vi "ReadLidarTesting.vi"() -> ()   [LabVIEW 2014]
uses:
  <instrlib>/Hokuyo URG Series/Public/Initialize-Standard.vi
  <instrlib>/Hokuyo URG Series/Hokuyo URG Series.lvlib
  <vilib>/robotics/Obstacle Avoidance/Advanced Vector Field Histogram/NI_Robotics_Vector Field Histogram.lvlib
panel:
  out "32bit integer":i32
  out "x+y":dbl
  out "x*y":dbl
  in  "maximum heading change (rad)":dbl=1.5707963267948966
  out "Meter":dbl(knob) scale=3.14..-3.14
  out "Waveform Graph":dbl[](graph)
  out "chosen heading (rad)":dbl
  in  "obstacle clearance distance":dbl
  in  "heading":T1
  in  "thresholds":T2
  out "XY Graph":cluster{"X":dbl[], "Y":dbl[]}(graph)
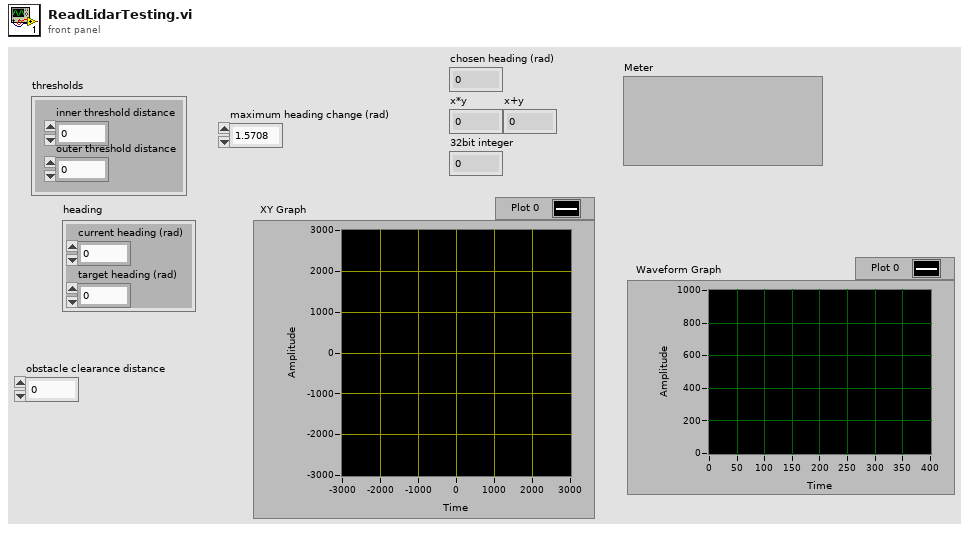
[diagram p1: front panel]
types:
  T1 = cluster{"current heading (rad)":dbl, "target heading (rad)":dbl}
  T2 = cluster{"inner threshold distance":dbl, "outer threshold distance":dbl}
  T3 = cluster{"Magnitude":u16[], "Direction":fxp<+/-,16,8>[]}
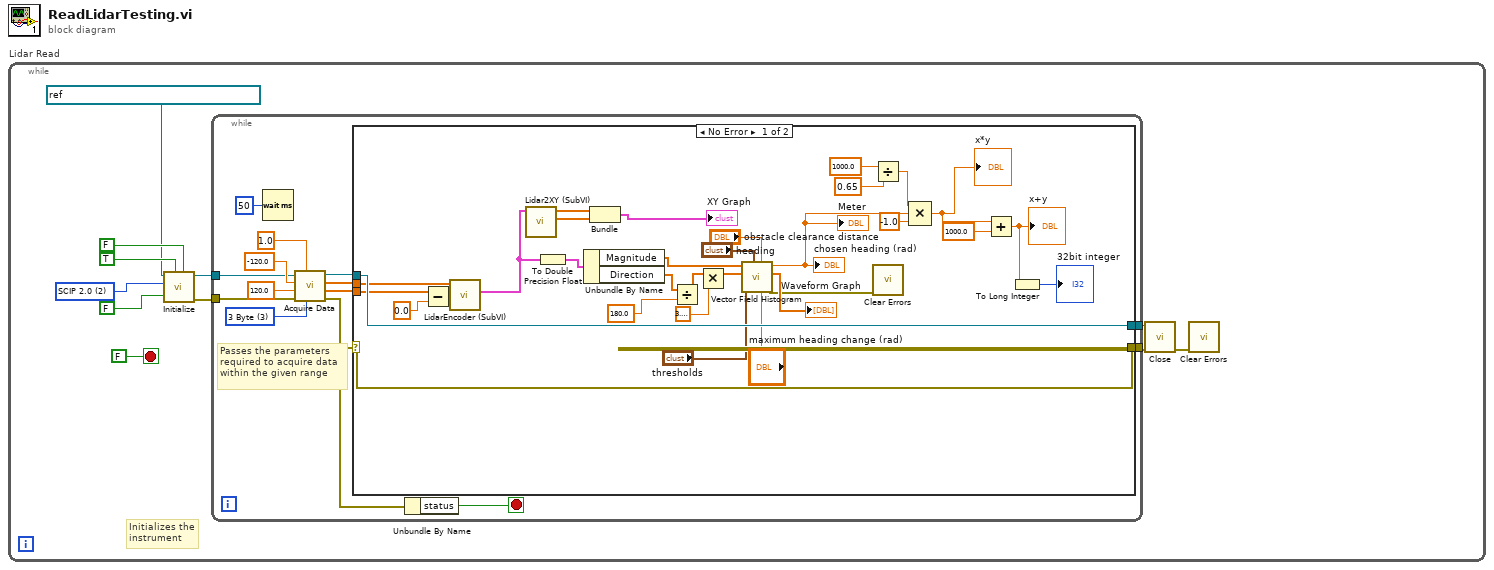
[diagram p0: block diagram]
diagram:
  n1 = while "Lidar Read" {
    stop <- FALSE stop-if-true
    w7 = u32 2 items=["Convert to Latest", "SCIP 1.1", "SCIP 2.0"] ("Protocol")
    # "Initializes the instrument"
    n2 = call-poly <instrlib>:"Initialize.vi"("Reset? (F: No)"=FALSE ("Reset Instrument (Disabled)"), "Checksum (Disabled)"=FALSE ("Checksum"), "ID Query? (Enabled)"=TRUE ("ID Query?"), "Protocol (2: SCIP 2.0)"=w7, "VISA resource name"=refnum<visa-resource-name> "TCPIP::192.168.0.10::10940::SOCKET") -> ("error out"=w4:errorcluster, "VISA resource name out"=w5:refnum<visa-resource-name>)  [unwired: 5 in]
    n3 = while {
      tunnel: w5 -> [w16]
      tunnel: [w25] -> w11
      tunnel: [w24] -> w6
      tunnel: w4 -> [w15]
      stop <- w12 stop-if-true
      w14 = u16 3 items=["2 Byte"=2, "3 Byte"=3] ("Encoding Width")
      # "Passes the parameters\nrequired to acquire data\nwithin the given range"
      n4 = Wait (ms)(milliseconds to wait=u32 50) -> ()  [unwired: 1 out]
      n5 = call <instrlib>:"Acquire Data.vi"("Data Encoding Width (3 Byte)"=w14, "Cluster Count (1)"=1.0 ("Cluster Count"), "error in (no error)"=w15, "End Point (120°)"=120.0 ("End Point"), "Start Point (-120°)"=-120.0 ("Start Point"), "VISA resource name"=w16) -> ("error out"=w20:errorcluster, "Direction"=w21:dbl[], "Magnitude"=w22:dbl[], "VISA resource name out"=w23:refnum<visa-resource-name>)  [unwired: 2 in]
      n6 = case shown="No Error" w20 {
        selector: w20 -> [w56 w59]
        tunnel: [w56 w59] -> w25
        tunnel: w23 -> [w57 w58]
        tunnel: [w57 w58] -> w24
        tunnel: w22 -> [w55 _]
        tunnel: w21 -> [w54 _]
        frame No Error {
          n7 = Subtract(x=w54, y=0.0) -> (x-y=w53:dbl[])
          n8 = call "LidarEncoder (SubVI).vi"("Direction"=w53, "Magnitude"=w55) -> ("Encoded"=w48:T3)  [unwired: 9 in]
          n9 = call "Lidar2XY (SubVI).vi"("Lidar"=w48) -> ("Y"=w50:dbl[], "X"=w51:dbl[])  [unwired: 9 in]
          n10 = To Double Precision Float(number=w48) -> (double precision float=w47:cluster{"Magnitude":dbl[], "Direction":dbl[]})
          n11 = Unbundle By Name(w47) -> ("Magnitude"=w46:dbl[], "Direction"=w44:dbl[])
          n12 = Bundle("X"=w51, "Y"=w50) -> (→"XY Graph":cluster{"X":dbl[], "Y":dbl[]})  [unwired: 1 in]
          n13 = Divide(x=w44, y=180.0) -> (x/y=w45:dbl[])
          n14 = Multiply(x=w45, y=3.141592653589793) -> (x*y=w42:dbl[])
          n15 = call <vilib>:"Vector Field Histogram.vi"("maximum heading change (rad)"="maximum heading change (rad)", "obstacle clearance distance"="obstacle clearance distance", "heading"="heading", "thresholds"="thresholds", "direction angles (rad)"=w42, "distances"=w46) -> ("error out"=w36:errorcluster, "histogram"=→"Waveform Graph":dbl[], "chosen heading (rad)"=w31:dbl)  [unwired: 2 in, 1 out]
          "chosen heading (rad)" <- w31
          "Meter" <- w31
          n16 = Divide(x=1000.0, y=0.65) -> (x/y=w34:dbl)
          n17 = call <vilib>:"Clear Errors.vi"("error in (no error)"=w36) -> ()  [unwired: 5 in, 2 out]
          n18 = Compound Arithmetic op=MULTIPLY(w34, w31, -1.0 ("value")) -> (w30:dbl)
          "x*y" <- w30
          n19 = Add(x=w30, y=1000.0) -> (x+y=w27:dbl)
          "x+y" <- w27
          n20 = To Long Integer(number=w27) -> (32bit integer=→"32bit integer":i32)
        }
        frame Error {
        }
      }
      n21 = Unbundle By Name(w20) -> ("status"=w12:bool)
    }
    n22 = call <instrlib>:"Close.vi"("error in (no error)"=w11, "VISA resource name"=w6) -> ("error out"=w1:errorcluster)  [unwired: 9 in]
    n23 = call <vilib>:"Clear Errors.vi"("error in (no error)"=w1) -> ()  [unwired: 5 in, 2 out]
  }
